vi "Publis Data to subscrtibers.vi"(8 "error in (no error)":errorcluster, 10 "Message Data":variant, 11 "RSeries_CAM in":refnum<class "RSeries_CAM.lvclass">) -> (0 "error out":errorcluster, 3 "RSeries_CAM out":refnum<class "RSeries_CAM.lvclass">)   [LabVIEW 2024, in "RSeries_CAM.lvlib" / "RSeries_CAM.lvclass"]
uses:
  RSeries_CAM.lvclass
  RSeries_CAM.lvclass/RSeries_CAM.ctl
  ARCH/Message Queue/Message Cluster.ctl
  ARCH/Message Queue/Message Queue.lvlib
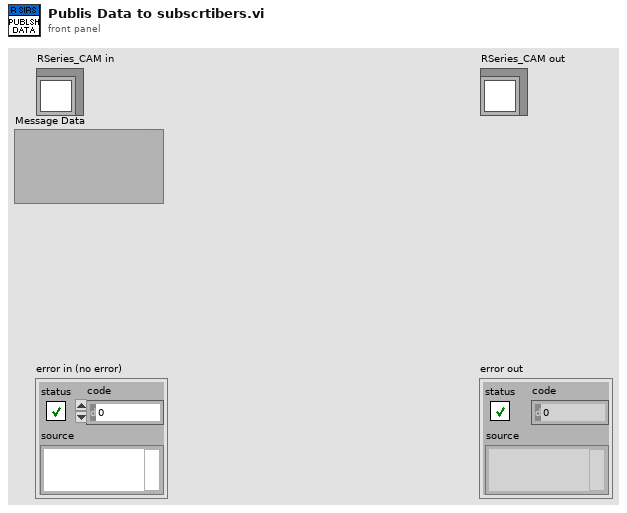
[diagram p1: front panel]
types:
  T1 = typedef "Message Queue.lvlib/Message Cluster.ctl" = cluster{"Message":string, "Message Data":variant}
  T2 = cluster{"Subscriber message":string, "Subscriber queue":refnum<queue>}[]
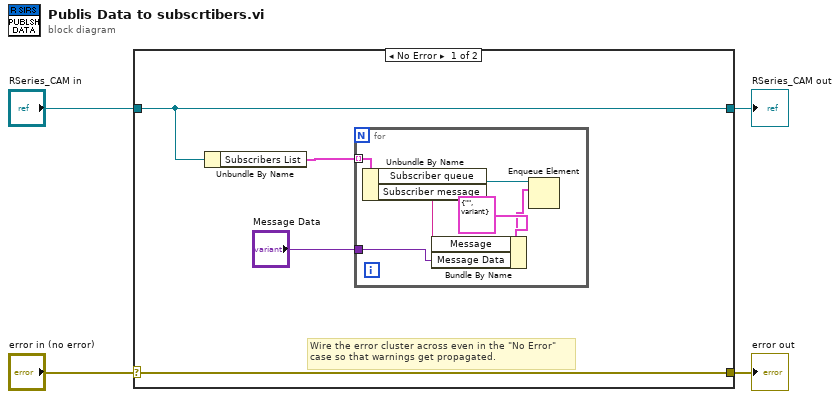
[diagram p0: block diagram]
diagram:
  n1 = case shown="No Error" "error in (no error)" {
    selector: "error in (no error)" -> [w8 w16]
    tunnel: [w8 w16] -> w3
    tunnel: [w7 w15] -> w1
    tunnel: "RSeries_CAM in" -> [w7 w15]
    frame No Error {
      # "Wire the error cluster across even in the \"No Error\"\ncase so that warnings get propagated."
      n2 = Unbundle By Name(w7) -> ("Subscribers List"=w6:T2)
      n3 = for {
        tunnel: w6 -> [w14] mode=indexing
        tunnel: "Message Data" -> [w9]
        n4 = Unbundle By Name(w14) -> ("Subscriber queue"=w13:refnum<queue>, "Subscriber message"=w11:string)
        n5 = Bundle By Name(cluster=T1 {"Message"="", "Message Data"=variant} ("element"), "Message"=w11, "Message Data"=w9) -> (w10:T1)
        n6 = Enqueue Element(queue=w13, element=w10) -> ()  [unwired: 2 in, 3 out]
      }
    }
    frame Error {
    }
  }
  "error out" <- w3
  "RSeries_CAM out" <- w1
